vi "readAnalysisOutput.vi"() -> (1 "bottle number":i64[](array[numeric]), 2 "fly number":i64[](array[numeric]), 3 "folder exists":bool, 4 "bottle label":string[](array[string]))   [LabVIEW 2012]
uses:
  image acquisition/GlobalBaslerCamera.vi
  <vilib>/Utility/file.llb/Read From Spreadsheet File (string).vi
  <vilib>/Utility/file.llb/Read From Spreadsheet File (I64).vi
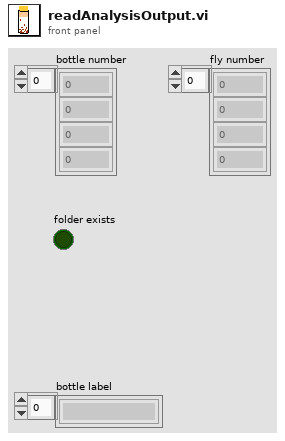
[diagram p1: front panel]
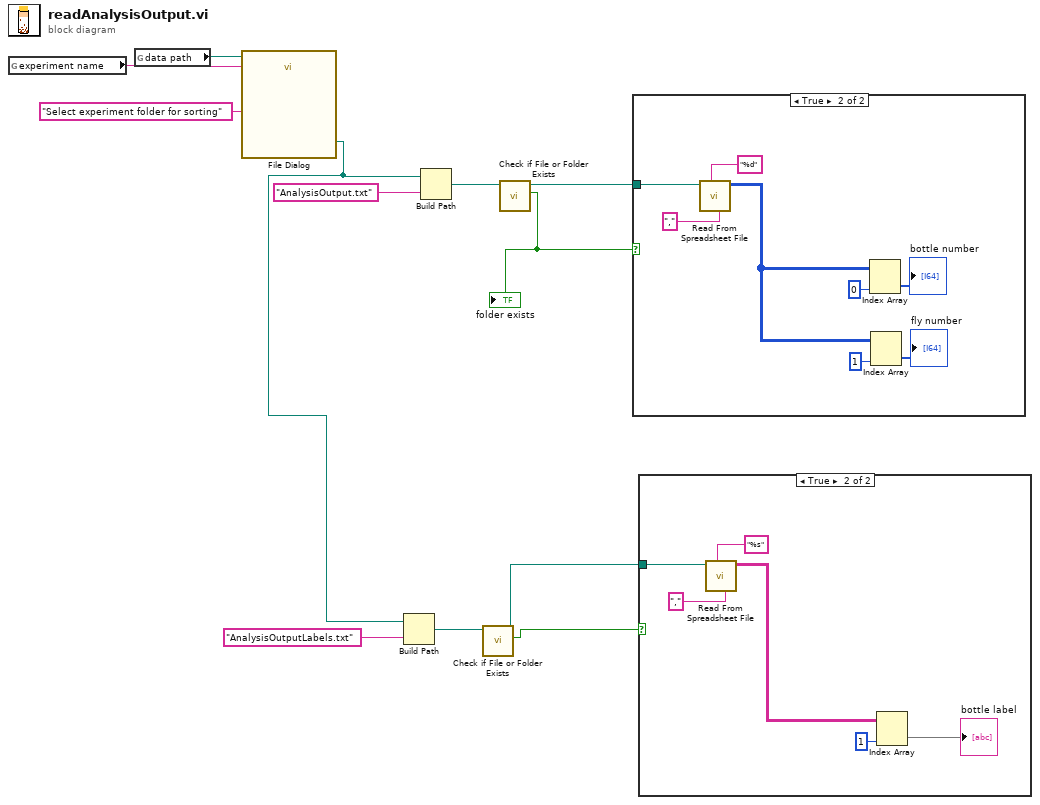
[diagram p0: block diagram]
diagram:
  n1 = global read "GlobalBaslerCamera.vi" "experiment name"() -> (w10:string)
  n2 = global read "GlobalBaslerCamera.vi" "data path"() -> (w12:path)
  n3 = call "File Dialog"("start path"=w12, "prompt"="Select experiment folder for sorting", "default name"=w10) -> ("selected path"=w3:path)  [unwired: 9 in, 3 out]
  n4 = Build Path(base path=w3, name or relative path="AnalysisOutputLabels.txt" ("string")) -> (appended path=w4:path)
  n5 = Build Path(base path=w3, name or relative path="AnalysisOutput.txt" ("string")) -> (appended path=w8:path)
  n6 = call <vilib>:"Check if File or Folder Exists.vi"("path"=w4) -> ("file or folder exists?"=w2:bool, "dup path"=w1:path)  [unwired: 8 in, 1 out]
  n7 = call <vilib>:"Check if File or Folder Exists.vi"("path"=w8) -> ("file or folder exists?"=w6:bool, "dup path"=w7:path)  [unwired: 8 in, 1 out]
  "folder exists" <- w6
  n8 = case shown="True" w6 {
    tunnel: w7 -> [_ w13]
    frame False {
    }
    frame True {
      n9 = call-poly <vilib>:"Read From Spreadsheet File.vi"("delimiter (\\t)"="," ("delimiter (\\t)"), "format (%d)"="%d", "file path (dialog if empty)"=w13) -> ("all rows"=w14:i64[][])  [unwired: 4 in, 4 out]
      n10 = Index Array(array=w14, index (col)=0 ("disabled index (col)")) -> (element=→"bottle number":i64[])  [unwired: 1 in]
      n11 = Index Array(array=w14, index (col)=1 ("disabled index (col)")) -> (element=→"fly number":i64[])  [unwired: 1 in]
    }
  }
  n12 = case shown="True" w2 {
    tunnel: w1 -> [_ w21]
    frame False {
    }
    frame True {
      n13 = call-poly <vilib>:"Read From Spreadsheet File.vi"("delimiter (\\t)"="," ("delimiter (\\t)"), "format (%s)"="%s" ("format (%d)"), "file path (dialog if empty)"=w21) -> ("all rows"=w22:string[][])  [unwired: 4 in, 4 out]
      n14 = Index Array(array=w22, index (col)=1 ("disabled index (col)")) -> (element=→"bottle label":string[])  [unwired: 1 in]
    }
  }
